vi "test_tape_nav.vi"() -> ()   [LabVIEW 2018]
uses:
  tape_counts.ctl
  <vilib>/Platform/TimedLoop/XDataNode/timing_clust.ctl
  <vilib>/Platform/TimedLoop/XDataNode/nitl_modes.ctl
  <vilib>/Platform/TimedLoop/XDataNode/wakeup.ctl
  validated_u32.ctl
  <vilib>/rvi/Emulation/niFpgaGetClockAttributes.vi
  <vilib>/rvi/Emulation/niFpgaSctlEmulationGetInTimedLoop.vi
  <vilib>/rvi/Emulation/niFpgaEmulationReportErrorSimple.vi
  <vilib>/rvi/Emulation/niFpgaEmulationIsFPGAContextNoSignature.vi
  <vilib>/rvi/DataTransferAndStorage/Container/Common/niFpgaContainerGetUniqueNameForEmu.vi
  <vilib>/rvi/Memory/Memory_Emulation/niFpgaMemoryEmulationCacheClearOnFirstRun.vi
  <vilib>/rvi/Memory/Memory_Emulation/nirvimemoryEmulationManagerCache_MakeExclusive.vi
  <vilib>/rvi/Memory/Memory_Emulation/niFpgaMemoryEmulationValidateCache.vi
  <vilib>/rvi/Memory/Memory_Emulation/nirvimemoryEmulationManagerCache_InsertValue.vi
  <vilib>/Utility/error.llb/Clear Errors.vi
  <vilib>/rvi/Memory/Memory_Emulation/nirvimemoryEmulationManagerCache_ReleaseExclusive.vi
  <vilib>/rvi/Memory/Memory_Emulation/nirvimemoryEmulationManagerCache_GetValue.vi
  <vilib>/rvi/Memory/Memory_Emulation/nirvimemoryEmulationManagerCache_SetValue.vi
  <vilib>/rvi/Emulation/niFpgaProcessEmulError.vi
  <vilib>/rvi/Emulation/niFpgaCriticalErrorInLSC.vi
  <vilib>/rvi/DataTransferAndStorage/Container/XNode/niFpgaContainer.xnode
  <vilib>/rvi/DataTransferAndStorage/Register/Emulation/niFpgaRegisterEmulation.vi
  <vilib>/Platform/TimedLoop/XDataNode/XDataNode.xnode
  <vilib>/Platform/TimedLoop/XDataNode/XDNodeRunTimeDep.lvlib
panel:
  in  "r":bool
  in  "l":bool
  in  "br":bool
  in  "bl":bool
  in  "stop":bool
  in  "light_sensor_window":u32
  in  "reset_tape":bool
  out "timestamp":fxp<+,48,41>
  out "Cluster":T1
  out "tape_detected":bool
  out "tape_count":u8
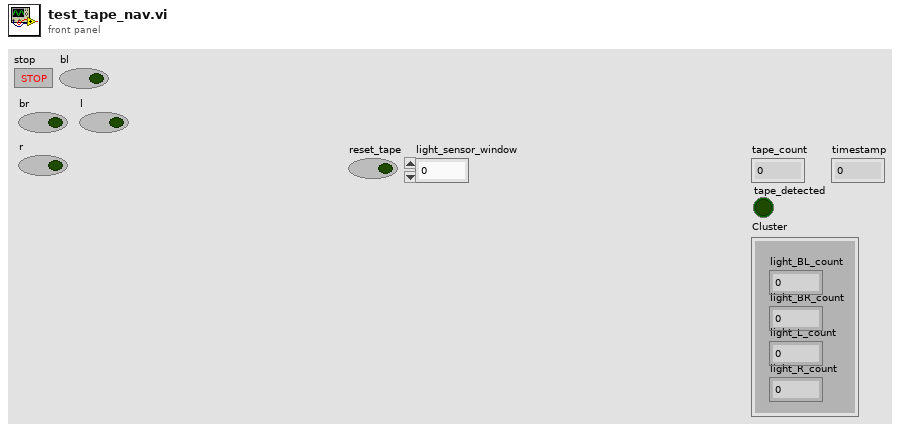
[diagram p1: front panel]
types:
  T1 = typedef "tape_counts.ctl" = cluster{"light_R_count":u8, "light_L_count":u8, "light_BR_count":u8, "light_BL_count":u8}
  T2 = typedef "XDNodeRunTimeDep.lvlib/timing_clust.ctl" = cluster{"Expected End [f-1]":u64, "Actual End [f-1]":u64, "Finished Late? [f-1]":bool, "Expected End [i-1]":u64, "Actual End [i-1]":u64, "Finished Late? [i-1]":bool, "Expected Start [i]":u64, "Actual Start [i]":u64, "Expected Start [f]":u64, "Actual Start [f]":u64, "Source Name":string, "Structure Name":string, "Period":i64, "Deadline":i64, "Offset":i64, "Start":i64, "Priority":i32, "Timeout":i32, "Mode":T3, "Wakeup Reason":T4, "Error":errorcluster, "Source Type":string, "Secondary Source Type":string, "Global End Time":u64, "Global Start Time":u64, "Frame Duration":u64, "Iteration Duration":u64, "Assigned CPU":i32, "I/O Scan Engine Mode":u32}
  T3 = typedef "XDNodeRunTimeDep.lvlib/nitl_modes.ctl" = enum32{"No Change", "Process missed periods, maintain original phase", "Discard missed periods, maintain original phase", "Process missed periods, ignore original phase", "Discard missed periods, ignore original phase"}
  T4 = typedef "XDNodeRunTimeDep.lvlib/wakeup.ctl" = enum32{"Normal", "Aborted", "Asynchronous wakeup", "Timing source error", "Timed loop error", "Timeout"}
  T5 = typedef "validated_u32.ctl" = cluster{"valid":bool, "value":u32}
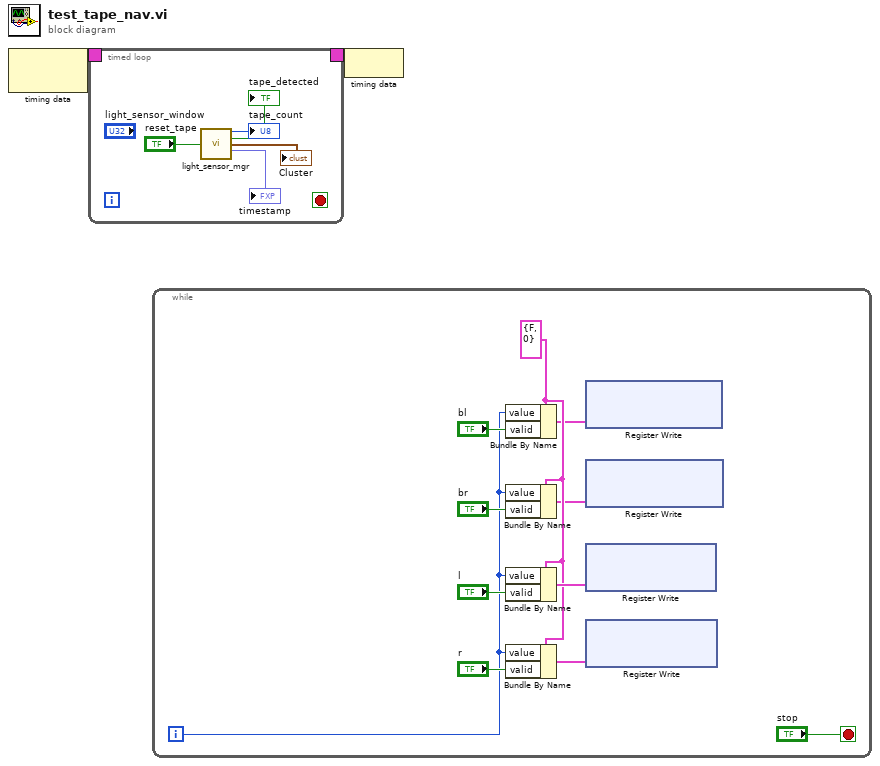
[diagram p0: block diagram]
diagram:
  n1 = node-c288() -> (w2:T2)  [unwired: 1 in]
  n2 = timed-loop {
    timing: w2 -> [_]
    timing-out: [_] -> w1
    stop <- _ stop-if-true
    n3 = call <userlib>:"light_sensor_mgr.vi"("reset_tape"="reset_tape") -> ("tape_count"=→"tape_count":u8, "tape_detected"=→"tape_detected":bool, "Cluster"=→"Cluster":T1, "timestamp"=→"timestamp":fxp<+,48,41>)  [unwired: 11 in]
  }
  n4 = while {
    i -> [w10]
    stop <- "stop" stop-if-true
    w17 = T5 {"valid"=FALSE, "value"=0} ("Cluster")
    n5 = Bundle By Name(cluster=w17, "value"=w10, "valid"="bl") -> (w15:T5)
    n6 = Bundle By Name(cluster=w17, "value"=w10, "valid"="br") -> (w16:T5)
    n7 = Bundle By Name(cluster=w17, "value"=w10, "valid"="l") -> (w18:T5)
    n8 = Bundle By Name(cluster=w17, "value"=w10, "valid"="r") -> (w19:T5)
    n9 = xnode "Register Write"("Data"=w15) -> ()  [unwired: 1 in, 1 out]
    n10 = xnode "Register Write"("Data"=w16) -> ()  [unwired: 1 in, 1 out]
    n11 = xnode "Register Write"("Data"=w18) -> ()  [unwired: 1 in, 1 out]
    n12 = xnode "Register Write"("Data"=w19) -> ()  [unwired: 1 in, 1 out]
  }
  n13 = node-c288(w1) -> ()
